vi "2pparameters.vi"(1 "Params in":T2={"Xpixels"=0, "Vxminref"=0.0, "Vxmaxref"=0.0, "P"=0.0, "Ypixels"=0, "Vyminref"=0.0, "Vymaxref"=0.0, "srate"=0.0, "sAOxy"=0, "timeout"=0.0, "type"="", "date"="", "time"="", "Colormap"=0, "Drawing Mode"=0, "Scanning Mode"=0, "square pixels"=FALSE, "square matrix"=FALSE, "Xpixels Img"=0, "Vx-min Img"=0.0, "VX-max Img"=0.0, "Ypixels Img"=0, "Vy-min Img"=0.0, "Vy-max Img "=0.0, "Angle Img"=0.0, "autoshutter"=FALSE, "finite"=FALSE, "cont"=FALSE, "wavdet"=FALSE, "measpoints"=0, "avpp"=0, "bufferAO"=0, "bufferAI"=0, "starttick"=0, "waveform"=path "", "Vx-ref"=0.0, "Vy-ref"=0.0, "refreshrate"=0.0, "refreshbuffer"=0, "tt_cycles"=0, "motorref"=refnum, "mirrorswitch"=refnum, "sample mode"=10123, "maxbufferAI"=0, "srateAODO"=0.0, "bin"=0.0, "Pel"=0.0, "Angle draw"=0.0, "srate Img"=0.0, "ROIimg_plotbounds"={"Left"=0, "Top"=0, "Right"=0, "Bottom"=0}, "auto OD"=FALSE, "ODfilt"=1, "aAI"=[], "aCI"=[], "aAO"=[], "aDO"=[], "refwfsize"=0.0, "Lifetime"=FALSE, "Vz-Img"=0.0, "Vz-ref"=0.0, "Vz-reset"=0.0, "AIoverride"=FALSE, "aAS"=[], "XYZstart"=[]} {"ODfilt" items=["OD 0"=1, "OD 0.5"=2, "OD 1"=3, "OD 2"=4, "OD 3"=5, "OD 4"=6]; "Scanning Mode" items=["Raster", "Spiral", "resonant"]; "Drawing Mode" items=["Image", "Fill Rectangle", "Fill Circle", "Draw Freeform", "Fill Freeform", "Ellipse", "Line"]; "maxbufferAI" min=-9 max=10; "sample mode" items=["Finite Samples"=10178, "Continuous Samples"=10123, "Hardware Timed Single Point"=12522]; "tt_cycles" min=-9 max=10; "refreshbuffer" min=-9 max=10; "refreshrate" min=-9.5 max=9.5; "Vx-ref" min=-9.5 max=9.5; "Vy-ref" min=-9.5 max=9.5; "bufferAI" min=0 step=1; "bufferAO" min=0 step=1; "avpp" min=0 step=1; "measpoints" step=1; "Vy-min Img" min=-9.5 max=9.5; "Ypixels Img" min=0 step=1; "Vx-min Img" min=-9.5 max=9.5; "Xpixels Img" min=0 step=1; "Colormap" items=["Grey", "Red", "Green", "Blue", "Hot", "Winter", "Jet"]; "Vyminref" min=-9.5 max=9.5; "Ypixels" min=0 step=1; "Vxminref" min=-9.5 max=9.5; "Xpixels" min=0 step=1}, 2 "command":string) -> (0 "params out":T2={"Xpixels"=0, "Vxminref"=0.0, "Vxmaxref"=0.0, "P"=0.0, "Ypixels"=0, "Vyminref"=0.0, "Vymaxref"=0.0, "srate"=0.0, "sAOxy"=0, "timeout"=0.0, "type"="", "date"="", "time"="", "Colormap"=0, "Drawing Mode"=0, "Scanning Mode"=0, "square pixels"=FALSE, "square matrix"=FALSE, "Xpixels Img"=0, "Vx-min Img"=0.0, "VX-max Img"=0.0, "Ypixels Img"=0, "Vy-min Img"=0.0, "Vy-max Img "=0.0, "Angle Img"=0.0, "autoshutter"=FALSE, "finite"=FALSE, "cont"=FALSE, "wavdet"=FALSE, "measpoints"=0, "avpp"=0, "bufferAO"=0, "bufferAI"=0, "starttick"=0, "waveform"=path "", "Vx-ref"=0.0, "Vy-ref"=0.0, "refreshrate"=0.0, "refreshbuffer"=0, "tt_cycles"=0, "motorref"=refnum, "mirrorswitch"=refnum, "sample mode"=10123, "maxbufferAI"=0, "srateAODO"=0.0, "bin"=0.0, "Pel"=0.0, "Angle draw"=0.0, "srate Img"=0.0, "ROIimg_plotbounds"={"Left"=0, "Top"=0, "Right"=0, "Bottom"=0}, "auto OD"=FALSE, "ODfilt"=1, "aAI"=[], "aCI"=[], "aAO"=[], "aDO"=[], "refwfsize"=0.0, "Lifetime"=FALSE, "Vz-Img"=0.0, "Vz-ref"=0.0, "Vz-reset"=0.0, "AIoverride"=FALSE, "aAS"=[], "XYZstart"=[]} {"ODfilt" items=["OD 0"=1, "OD 0.5"=2, "OD 1"=3, "OD 2"=4, "OD 3"=5, "OD 4"=6]; "Scanning Mode" items=["Raster", "Spiral", "resonant"]; "Drawing Mode" items=["Image", "Fill Rectangle", "Fill Circle", "Draw Freeform", "Fill Freeform", "Ellipse", "Line"]; "maxbufferAI" min=-9 max=10; "sample mode" items=["Finite Samples"=10178, "Continuous Samples"=10123, "Hardware Timed Single Point"=12522]; "tt_cycles" min=-9 max=10; "refreshbuffer" min=-9 max=10; "refreshrate" min=-9.5 max=9.5; "Vx-ref" min=-9.5 max=9.5; "Vy-ref" min=-9.5 max=9.5; "bufferAI" min=0 step=1; "bufferAO" min=0 step=1; "avpp" min=0 step=1; "measpoints" step=1; "Vy-min Img" min=-9.5 max=9.5; "Ypixels Img" min=0 step=1; "Vx-min Img" min=-9.5 max=9.5; "Xpixels Img" min=0 step=1; "Colormap" items=["Grey", "Red", "Green", "Blue", "Hot", "Winter", "Jet"]; "Vyminref" min=-9.5 max=9.5; "Ypixels" min=0 step=1; "Vxminref" min=-9.5 max=9.5; "Xpixels" min=0 step=1})   [LabVIEW 2015]
uses:
  <vilib>/Utility/miscctls.llb/LVRectTypeDef.ctl
panel:
  # "Samples per image"
  # "active AI channels"
  # "active CI channels"
  # "active AO channels"
  # "active DO channels"
  # "active Autoshutter channels"
  # "position as measured at start"
  # "Samples per image"
  # "active AI channels"
  # "active CI channels"
  # "active AO channels"
  # "active DO channels"
  # "active Autoshutter channels"
  # "position as measured at start"
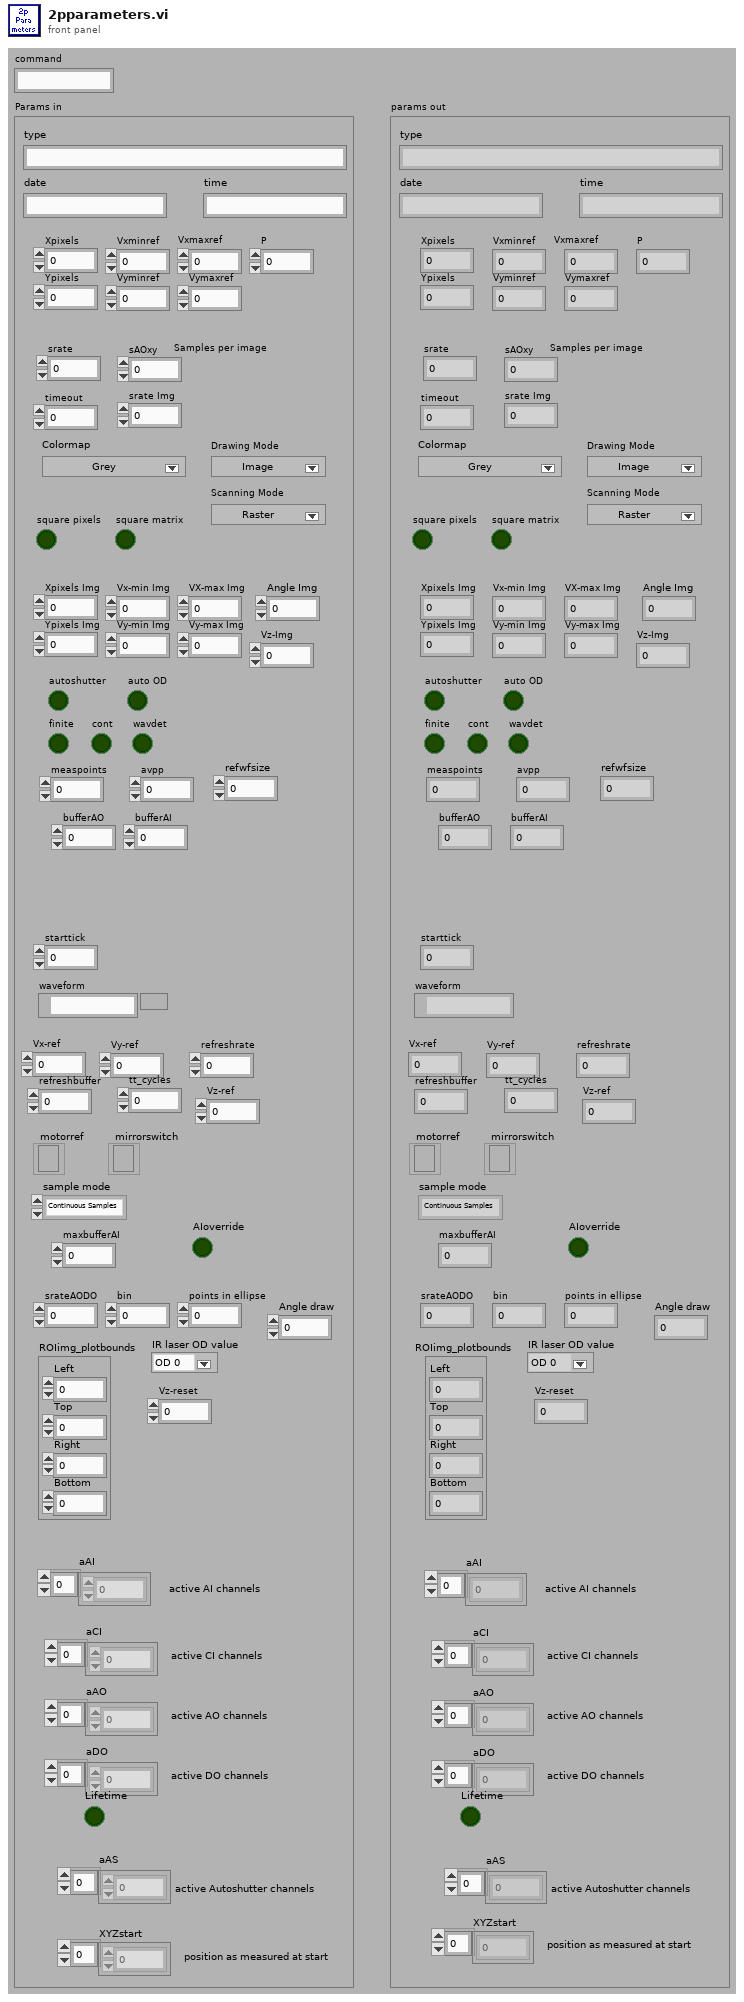
[diagram p1: front panel]
types:
  T1 = typedef "LVRectTypeDef.ctl" = cluster{"Left":i16, "Top":i16, "Right":i16, "Bottom":i16}
  T2 = cluster{"Xpixels":i32, "Vxminref":dbl, "Vxmaxref":dbl, "P":dbl, "Ypixels":i32, "Vyminref":dbl, "Vymaxref":dbl, "srate":sgl, "sAOxy":i32, "timeout":dbl, "type":string, "date":string, "time":string, "Colormap":u16, "Drawing Mode":u16, "Scanning Mode":u16, "square pixels":bool, "square matrix":bool, "Xpixels Img":i32, "Vx-min Img":dbl, "VX-max Img":dbl, "Ypixels Img":i32, "Vy-min Img":dbl, "Vy-max Img ":dbl, "Angle Img":dbl, "autoshutter":bool, "finite":bool, "cont":bool, "wavdet":bool, "measpoints":i32, "avpp":i32, "bufferAO":i32, "bufferAI":i32, "starttick":u32, "waveform":path, "Vx-ref":dbl, "Vy-ref":dbl, "refreshrate":dbl, "refreshbuffer":i32, "tt_cycles":i32, "motorref":refnum<k7>, "mirrorswitch":refnum<k7>, "sample mode":i32, "maxbufferAI":i32, "srateAODO":sgl, "bin":sgl, "Pel":sgl, "Angle draw":dbl, "srate Img":sgl, "ROIimg_plotbounds":T1, "auto OD":bool, "ODfilt":u16, "aAI":i32[], "aCI":i32[], "aAO":u32[], "aDO":u32[], "refwfsize":dbl, "Lifetime":bool, "Vz-Img":dbl, "Vz-ref":dbl, "Vz-reset":dbl, "AIoverride":bool, "aAS":u32[], "XYZstart":dbl[]}
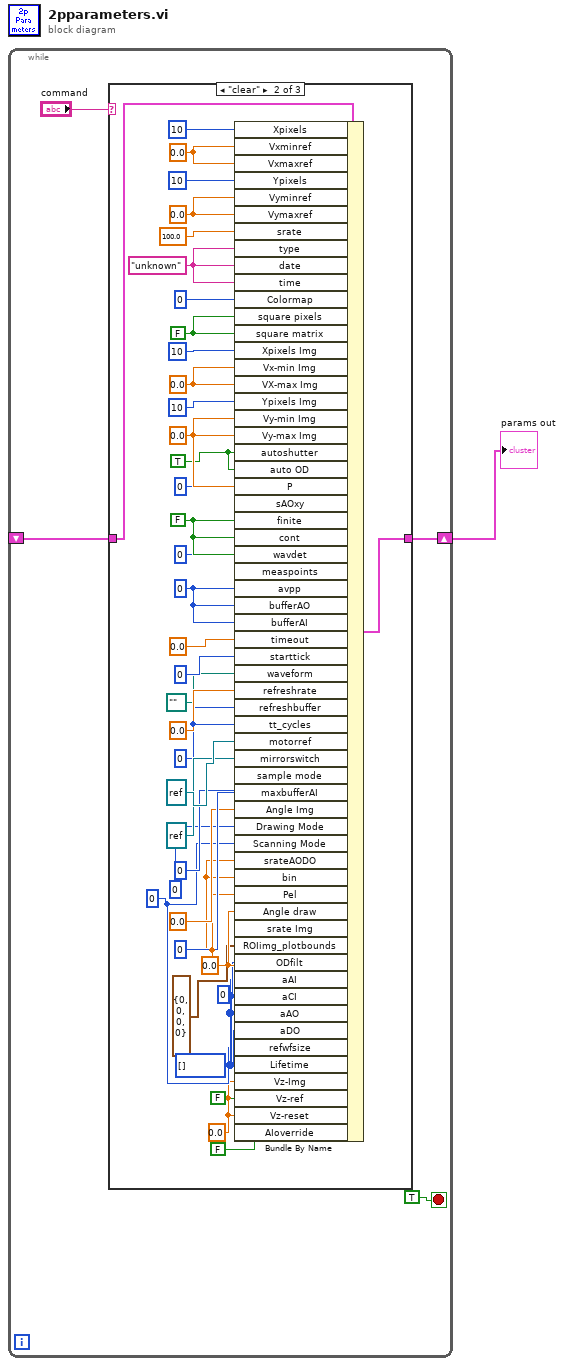
[diagram p0: block diagram]
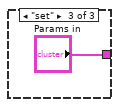
[diagram p3: hidden frame]
diagram:
  n1 = while {
    shift-right: [w3] -> w1
    shift-left: _ -> [w2]
    stop <- TRUE stop-if-true
    n2 = case shown="\"clear\"" "command" {
      tunnel: [w6 w43 "Params in"] -> w3
      tunnel: w2 -> [w6 w44 _]
      frame "get", Default {
      }
      frame "clear" {
        w8 = 0.0 ("Vz-ref")
        w11 = i32[] [] ("Active AI")
        w16 = sgl 0.0 ("srateAODO")
        w10 = u16 0 ("Scanning Mode")
        w17 = 0 ("tt_cycles")
        w19 = 0 ("sAOxy")
        w29 = FALSE ("finite")
        w14 = TRUE ("autoshutter")
        w33 = 0.0 ("Vy-max")
        w31 = 0.0 ("Vy-max")
        w35 = FALSE ("square pixels")
        w39 = 0.0 ("Vy-max")
        w40 = 0.0 ("Vy-max")
        w42 = "unknown" ("date")
        n3 = Bundle By Name(cluster=w44, "Xpixels"=10, "Vxminref"=w39, "Vxmaxref"=w39, "Ypixels"=10, "Vyminref"=w40, "Vymaxref"=w40, "srate"=100.0 ("AO rate"), "type"=w42, "date"=w42, "time"=w42, "Colormap"=u16 0, "square pixels"=w35, "square matrix"=w35, "Xpixels Img"=10 ("Xpixels"), "Vx-min Img"=w33, "VX-max Img"=w33, "Ypixels Img"=10 ("Ypixels"), "Vy-min Img"=w31, "Vy-max Img"=w31, "autoshutter"=w14, "auto OD"=w14, "P"=w31, "sAOxy"=0, "finite"=w29, "cont"=w29, "wavdet"=w29, "measpoints"=u32 0 ("sAOxy"), "avpp"=w19, "bufferAO"=w19, "bufferAI"=w19, "timeout"=0.0 ("Vy-max"), "starttick"=u32 0, "waveform"=path "", "refreshrate"=0.0, "refreshbuffer"=w17, "tt_cycles"=w17, "motorref"=refnum<k7> refnum, "mirrorswitch"=refnum<k7> refnum, "sample mode"=0, "maxbufferAI"=0, "Angle Img"=0.0 ("sampletreshold"), "Drawing Mode"=u16 0, "Scanning Mode"=w10, "srateAODO"=w16, "bin"=w16, "Pel"=w16, "Angle draw"=w16, "srate Img"=w16, "ROIimg_plotbounds"=T1 {"Left"=0, "Top"=0, "Right"=0, "Bottom"=0}, "ODfilt"=u16 0, "aAI"=w11, "aCI"=w11, "aAO"=w11, "aDO"=w11, "refwfsize"=w10, "Lifetime"=FALSE, "Vz-Img"=w8, "Vz-ref"=w8, "Vz-reset"=w8, "AIoverride"=FALSE) -> (w43:T2)
      }
      frame "set" {
      }
    }
  }
  "params out" <- w1
